vi "grSim Robot Command Decoder.vi"(8 "error in (no error)":errorcluster, 10 "Array":u8[](array[numeric]) format="%02x") -> (0 "error out":errorcluster, 1 "array w/ subset deleted":u8[](array[numeric]), 2 "Robot cluster":T1)   [LabVIEW 2016]
uses:
  grsim/grSim Robot Command.ctl
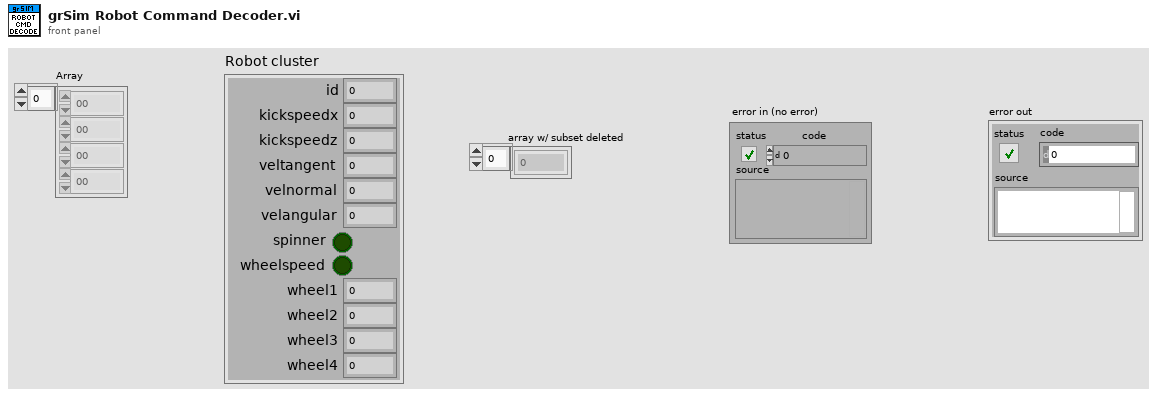
[diagram p1: front panel]
types:
  T1 = typedef "grSim Robot Command.ctl" = cluster{"id":u32, "kickspeedx":sgl, "kickspeedz":sgl, "veltangent":sgl, "velnormal":sgl, "velangular":sgl, "spinner":bool, "wheelspeed":bool, "wheel1":sgl, "wheel2":sgl, "wheel3":sgl, "wheel4":sgl}
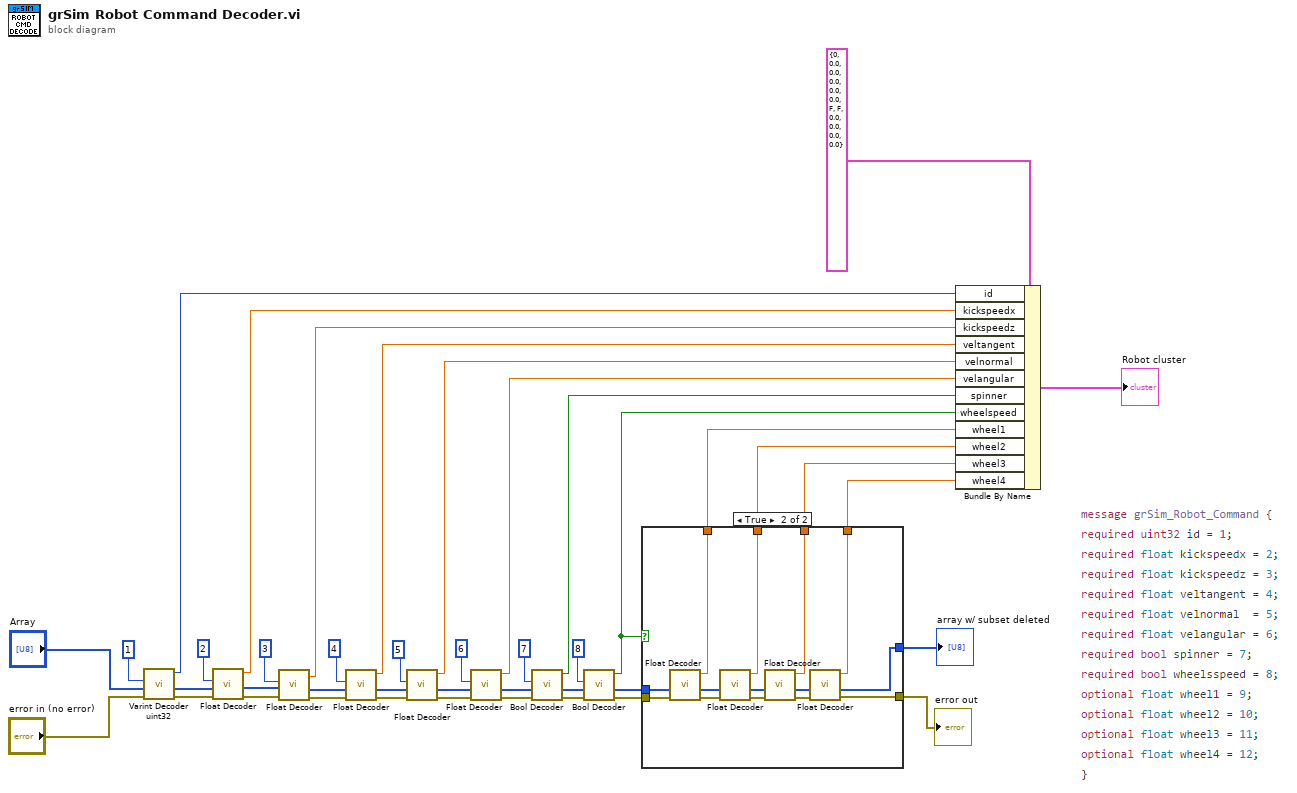
[diagram p0: block diagram]
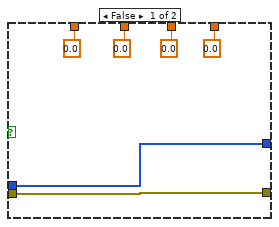
[diagram p2: hidden frame]
diagram:
  n1 = call "Varint Decoder uint32.vi"("error in (no error)"="error in (no error)", "Array"="Array", "Key"=1) -> ("error out"=w24:errorcluster, "array w/ subset deleted"=w33:u8[], "Varint"=w34:u32)  [unwired: 5 in, 1 out]
  n2 = call "Float Decoder.vi"("error in (no error)"=w24, "Array"=w33, "Key"=2) -> ("error out"=w23:errorcluster, "array w/ subset deleted"=w32:u8[], "Float"=w15:sgl)  [unwired: 5 in, 1 out]
  n3 = call "Float Decoder.vi"("error in (no error)"=w23, "Array"=w32, "Key"=3) -> ("error out"=w22:errorcluster, "array w/ subset deleted"=w31:u8[], "Float"=w14:sgl)  [unwired: 5 in, 1 out]
  n4 = call "Float Decoder.vi"("error in (no error)"=w22, "Array"=w31, "Key"=4) -> ("error out"=w21:errorcluster, "array w/ subset deleted"=w30:u8[], "Float"=w13:sgl)  [unwired: 5 in, 1 out]
  n5 = call "Float Decoder.vi"("error in (no error)"=w21, "Array"=w30, "Key"=5) -> ("error out"=w20:errorcluster, "array w/ subset deleted"=w29:u8[], "Float"=w12:sgl)  [unwired: 5 in, 1 out]
  n6 = call "Float Decoder.vi"("error in (no error)"=w20, "Array"=w29, "Key"=6) -> ("error out"=w19:errorcluster, "array w/ subset deleted"=w28:u8[], "Float"=w11:sgl)  [unwired: 5 in, 1 out]
  n7 = call "Bool Decoder.vi"("error in (no error)"=w19, "Array"=w28, "Key"=7) -> ("error out"=w18:errorcluster, "array w/ subset deleted"=w27:u8[], "bool"=w5:bool)  [unwired: 5 in, 1 out]
  n8 = call "Bool Decoder.vi"("error in (no error)"=w18, "Array"=w27, "Key"=8) -> ("error out"=w17:errorcluster, "array w/ subset deleted"=w26:u8[], "bool"=w2:bool)  [unwired: 5 in, 1 out]
  n9 = case shown="True" w2 {
    tunnel: w26 -> [w43 w62]
    tunnel: w17 -> [w48 w58]
    tunnel: [w48 w54] -> w16
    tunnel: [sgl 0.0 ("Float") w53] -> w10
    tunnel: [sgl 0.0 ("Float") w52] -> w9
    tunnel: [sgl 0.0 ("Float") w51] -> w8
    tunnel: [sgl 0.0 ("Float") w50] -> w7
    tunnel: [w43 w49] -> w3
    frame False {
    }
    frame True {
      n10 = call "Float Decoder.vi"("error in (no error)"=w58, "Array"=w62) -> ("error out"=w57:errorcluster, "array w/ subset deleted"=w61:u8[], "Float"=w53:sgl)  [unwired: 6 in, 1 out]
      n11 = call "Float Decoder.vi"("error in (no error)"=w57, "Array"=w61) -> ("error out"=w56:errorcluster, "array w/ subset deleted"=w60:u8[], "Float"=w52:sgl)  [unwired: 6 in, 1 out]
      n12 = call "Float Decoder.vi"("error in (no error)"=w56, "Array"=w60) -> ("error out"=w55:errorcluster, "array w/ subset deleted"=w59:u8[], "Float"=w51:sgl)  [unwired: 6 in, 1 out]
      n13 = call "Float Decoder.vi"("error in (no error)"=w55, "Array"=w59) -> ("error out"=w54:errorcluster, "array w/ subset deleted"=w49:u8[], "Float"=w50:sgl)  [unwired: 6 in, 1 out]
    }
  }
  "error out" <- w16
  "array w/ subset deleted" <- w3
  n14 = Bundle By Name(cluster=T1 {"id"=0, "kickspeedx"=0.0, "kickspeedz"=0.0, "veltangent"=0.0, "velnormal"=0.0, "velangular"=0.0, "spinner"=FALSE, "wheelspeed"=FALSE, "wheel1"=0.0, "wheel2"=0.0, "wheel3"=0.0, "wheel4"=0.0} ("grSim Robot Command"), "id"=w34, "kickspeedx"=w15, "kickspeedz"=w14, "veltangent"=w13, "velnormal"=w12, "velangular"=w11, "spinner"=w5, "wheelspeed"=w2, "wheel1"=w10, "wheel2"=w9, "wheel3"=w8, "wheel4"=w7) -> (→"Robot cluster":T1)
